vi "Get Master Slave Jog Velocity Scalling Coefficients.vi"(4 "error in (no error)":errorcluster, 7 "VISA resource name":refnum<visa-resource-name>) -> (0 "error out":errorcluster, 1 "B":dbl format="%.6g", 2 "A":dbl format="%.6g", 3 "VISA resource name out":refnum<visa-resource-name>)   [LabVIEW 2018, in "Newport ESP301.lvlib"]
doc: "Reads the jog velocity scalling coefficients for slave axis."
uses:
  Newport ESP301.lvlib
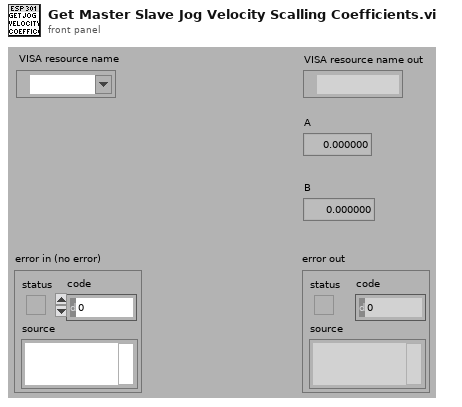
[diagram p1: front panel]
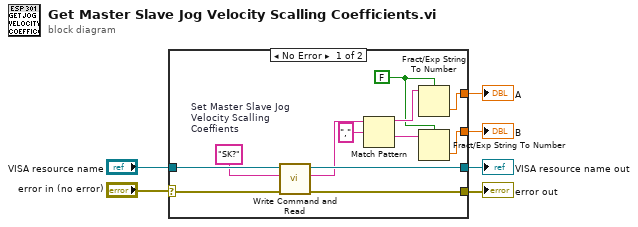
[diagram p0: block diagram]
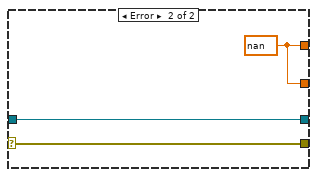
[diagram p2: hidden frame]
diagram:
  n1 = case shown="No Error" "error in (no error)" {
    selector: "error in (no error)" -> [w15 w21]
    tunnel: [w17 w21] -> w6
    tunnel: "VISA resource name" -> [w18 w20]
    tunnel: [w16 w20] -> w5
    tunnel: [w9 w19] -> w2
    tunnel: [w8 w19] -> w1
    frame No Error {
      w10 = FALSE ("utiliser le séparateur décimal du système (V)")
      w7 = "SK?"  # Set Master Slave Jog Velocity Scalling Coeffients
      n2 = call "Write Command and Read.vi"("error in (no error)"=w15, "Command"=w7, "VISA resource name"=w18) -> ("error out"=w17:errorcluster, "Returned string"=w14:string, "VISA resource name out"=w16:refnum<visa-resource-name>)  [unwired: 4 in]
      n3 = Match Pattern(string=w14, regular expression="," ("expression régulière")) -> (before substring=w12:string, after substring=w11:string)  [unwired: 1 in, 2 out]
      n4 = Fract/Exp String To Number(use system decimal point (T)=w10, string=w12) -> (number=w9:dbl)  [unwired: 2 in, 1 out]
      n5 = Fract/Exp String To Number(use system decimal point (T)=w10, string=w11) -> (number=w8:dbl)  [unwired: 2 in, 1 out]
    }
    frame Error {
      w19 = nan
    }
  }
  "error out" <- w6
  "VISA resource name out" <- w5
  "A" <- w2
  "B" <- w1
